vi "serverstreaming_client.vi"() -> ()   [LabVIEW 2019]
uses:
  Generated_client/RPC Messages/routeguide_Color.ctl
  Generated_client/RPC Messages/routeguide_request.ctl
  Generated_client/Generated_client.lvlib
panel:
  out "response_color":T1
  out "respo_message":string[](array[string])
  out "resp_numb":i32[](array[numeric])
  in  "request_color":T1
  in  "request_message":string
  in  "request_number":i32
  out "error out":errorcluster
  in  "error in":errorcluster
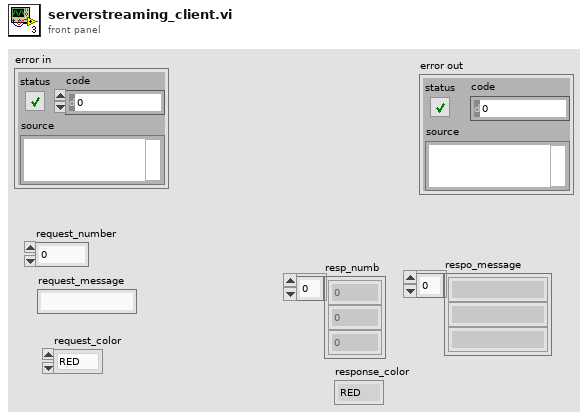
[diagram p1: front panel]
types:
  T1 = typedef "Generated_client.lvlib/routeguide_Color.ctl" = enum32{"RED", "GREEN", "BLUE"}
  T2 = typedef "Generated_client.lvlib/routeguide_request.ctl" = cluster{"request_number":i32, "request_message":string, "request_color":T1}
  T3 = typedef "grpc-lvsupport-release.lvlib/grpcId.ctl" = u64
  T4 = typedef "Generated_client.lvlib/routeguide_response.ctl" = cluster{"response_number":i32, "response_message":string, "response_color":T1}
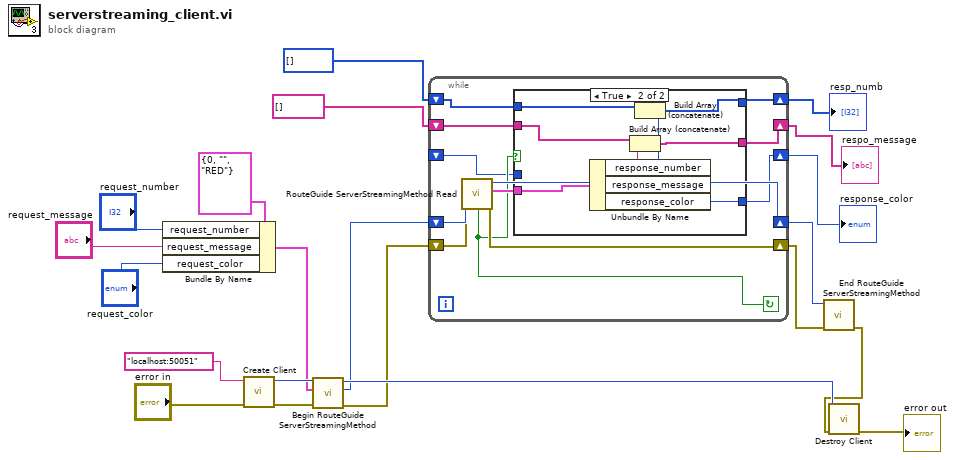
[diagram p0: block diagram]
diagram:
  n1 = Bundle By Name(cluster=T2 {"request_number"=0, "request_message"="", "request_color"=enum."RED"} ("routeguide_request"), "request_number"="request_number", "request_message"="request_message", "request_color"="request_color") -> (w14:T2)
  n2 = call "Create Client.vi"("error in"="error in", "address"="localhost:50051") -> ("error out"=w13:errorcluster, "gRPC ID Out"=w15:T3)  [unwired: 8 in]
  n3 = call "Begin RouteGuide ServerStreamingMethod.vi"("error in"=w13, "Request Data"=w14, "gRPC ID"=w15) -> ("error out"=w10:errorcluster, "Call Id Out"=w11:T3, "gRPC ID out"=w12:T3)  [unwired: 6 in]
  n4 = while {
    shift-right: [w32] -> w4
    shift-left: w11 -> [w33]
    shift-right: [w29] -> w3
    shift-left: w10 -> [w30]
    shift-right: [w27] -> w8
    shift-left: i32[] [] -> [w28]
    shift-right: [w25] -> w6
    shift-left: string[] [] -> [w26]
    shift-right: [w23] -> w1
    shift-left: _ -> [w22]
    stop <- w24 continue-if-true
    n5 = call "RouteGuide ServerStreamingMethod Read.vi"("error in"=w30, "Call ID in"=w33) -> ("error out"=w29:errorcluster, "Success"=w24:bool, "Response Data"=w31:T4, "Call ID"=w32:T3)  [unwired: 6 in]
    n6 = case shown="True" w24 {
      tunnel: w31 -> [_ w44]
      tunnel: w28 -> [w36 w42]
      tunnel: [w36 w41] -> w27
      tunnel: w26 -> [w35 w39]
      tunnel: [w35 w38] -> w25
      tunnel: [w34 w37] -> w23
      tunnel: w22 -> [w34 _]
      frame False {
      }
      frame True {
        n7 = Unbundle By Name(w44) -> ("response_number"=w43:i32, "response_message"=w40:string, "response_color"=w37:T1)
        n8 = Build Array (concatenate)(w39, w40) -> (w38:string[])
        n9 = Build Array (concatenate)(w42, w43) -> (w41:i32[])
      }
    }
  }
  "resp_numb" <- w8
  "respo_message" <- w6
  "response_color" <- w1
  n10 = call "End RouteGuide ServerStreamingMethod.vi"("error in"=w3, "Call ID in"=w4) -> ("error out"=w2:errorcluster)  [unwired: 8 in, 1 out]
  n11 = call "Destroy Client.vi"("error in"=w2, "gRPC ID"=w12) -> ("error out"=→"error out":errorcluster)  [unwired: 9 in]
